vi "Sequence Stop.vi"(1 "Sequencer Data Context IN":T1={"Sequencer State"=enum."Idle", "Event Timeout"=-1, "Current Index"=0, "Sequence Timeout"=0, "Turbine RPM Array"=[], "Pump RPM Array"=[], "Duration (Seconds) Array"=[], "Folder Path"=path ""}) -> (0 "Sequencer Data Context OUT":T1={"Sequencer State"=enum."Idle", "Event Timeout"=-1, "Current Index"=0, "Sequence Timeout"=0, "Turbine RPM Array"=[], "Pump RPM Array"=[], "Duration (Seconds) Array"=[], "Folder Path"=path ""})   [LabVIEW 2024, in "Auto Modo.lvlib"]
uses:
  Auto Modo.lvlib
  Sequencer Data Context.ctl
  Sequencer State.ctl
  Hardware Controller/Hardware Controller.lvlib
  Logger/Logger.lvlib
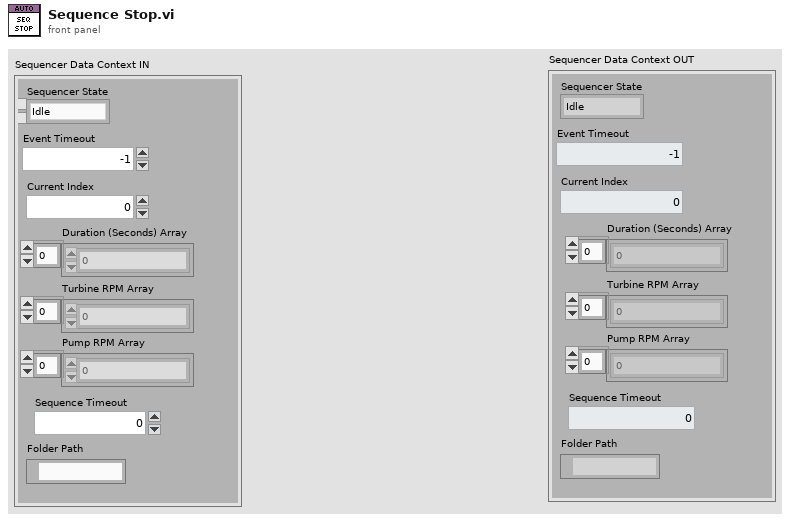
[diagram p1: front panel]
types:
  T1 = typedef "Auto Modo.lvlib/Sequencer Data Context.ctl" = cluster{"Sequencer State":T2, "Event Timeout":i32, "Current Index":i32, "Sequence Timeout":i32, "Turbine RPM Array":dbl[], "Pump RPM Array":dbl[], "Duration (Seconds) Array":dbl[], "Folder Path":path}
  T2 = typedef "Auto Modo.lvlib/Sequencer State.ctl" = enum16{"Idle", "Clear Drive Fault", "Check Drive Fault", "Set Ready to Switch ON", "Check Ready to Switch ON", "Enable Operation", "Check Enable Operation", "Set Drive RPM", "Check Drive RPM", "Next Drive RPM", "Final"}
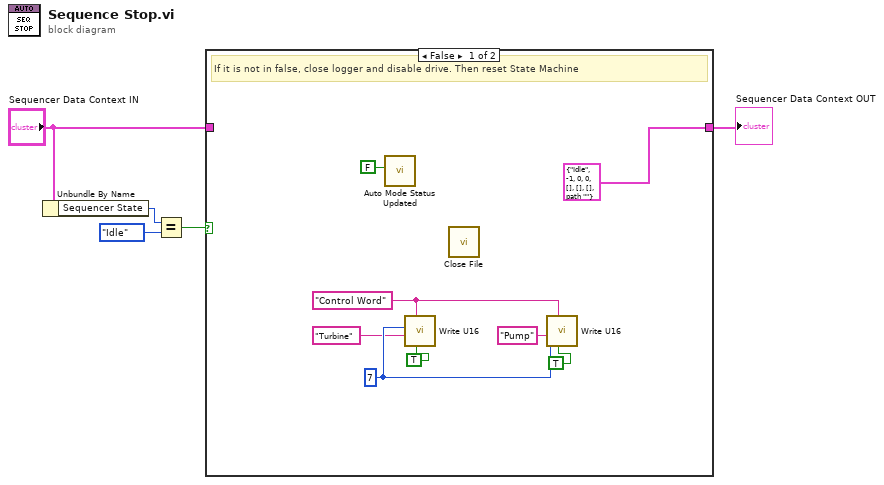
[diagram p0: block diagram]
diagram:
  n1 = Unbundle By Name("Sequencer Data Context IN") -> ("Sequencer State"=w5:T2)
  n2 = Equal?(x=w5, y=Sequencer_State."Idle") -> (x = y?=w3:bool)
  n3 = case shown="False" w3 {
    tunnel: [T1 {"Sequencer State"=enum."Idle", "Event Timeout"=-1, "Current Index"=0, "Sequence Timeout"=0, "Turbine RPM Array"=[], "Pump RPM Array"=[], "Duration (Seconds) Array"=[], "Folder Path"=path ""} ("Sequencer Data Context") w14] -> w1
    tunnel: "Sequencer Data Context IN" -> [_ w14]
    frame False {
      w11 = "Control Word" ("Variable")
      w9 = u16 7 ("Data")
      # "If it is not in false, close logger and disable drive. Then reset State Machine"
      n4 = call "Auto Mode Status Updated.vi"("Auto Mode?"=FALSE) -> ()  [unwired: 10 in, 1 out]
      n5 = call "Write U16.vi"("wait for reply (T)"=TRUE, "Variable"=w11, "Drive"="Turbine", "Data"=w9) -> ()  [unwired: 6 in, 2 out]
      n6 = call "Close File.vi"() -> ()  [unwired: 9 in, 3 out]
      n7 = call "Write U16.vi"("wait for reply (T)"=TRUE, "Variable"=w11, "Drive"="Pump", "Data"=w9) -> ()  [unwired: 6 in, 2 out]
    }
    frame True {
      # "If it is idling, do nothing"
    }
  }
  "Sequencer Data Context OUT" <- w1
